vi "Check Linux Partition Size.vi"(8 "Error In":errorcluster, 10 "Warnings":T1[](array[typedef]), 11 "Install LV Data":T2={"SSH Session"=refnum, "Status Log"="", "Detailed Log"="", "Credentials"={"Hostname or IP"="192.168.7.2", "Username"="root", "Password"=""}, "Target Info"={"OS Version"="", "CPU"="", "Systemd Version"="", "Internet Access"=FALSE, "Device Type"="", "LV Installed Ver"="", "LV Available Ver"="", "LV Upgrade Available"=FALSE, "Hostname"="", "NIC Info"=[]}, "Reboot Required?"=FALSE}) -> (0 "Error Out":errorcluster, 2 "Warnings":T1[](array[typedef]), 3 "Install LV Data":T2={"SSH Session"=refnum, "Status Log"="", "Detailed Log"="", "Credentials"={"Hostname or IP"="192.168.7.2", "Username"="root", "Password"=""}, "Target Info"={"OS Version"="", "CPU"="", "Systemd Version"="", "Internet Access"=FALSE, "Device Type"="", "LV Installed Ver"="", "LV Available Ver"="", "LV Upgrade Available"=FALSE, "Hostname"="", "NIC Info"=[]}, "Reboot Required?"=FALSE})   [LabVIEW 2020, in "LMH-LINX.lvlib"]
uses:
  LMH-LINX.lvlib
  Install LV Data.ctl
  Target Info.ctl
  NIC Info.ctl
  NIC Mode.ctl
  Target Compatibility Warnings.ctl
  BBB Expand File System.vi
  <vilib>/regexp/Match Regular Expression.xnode
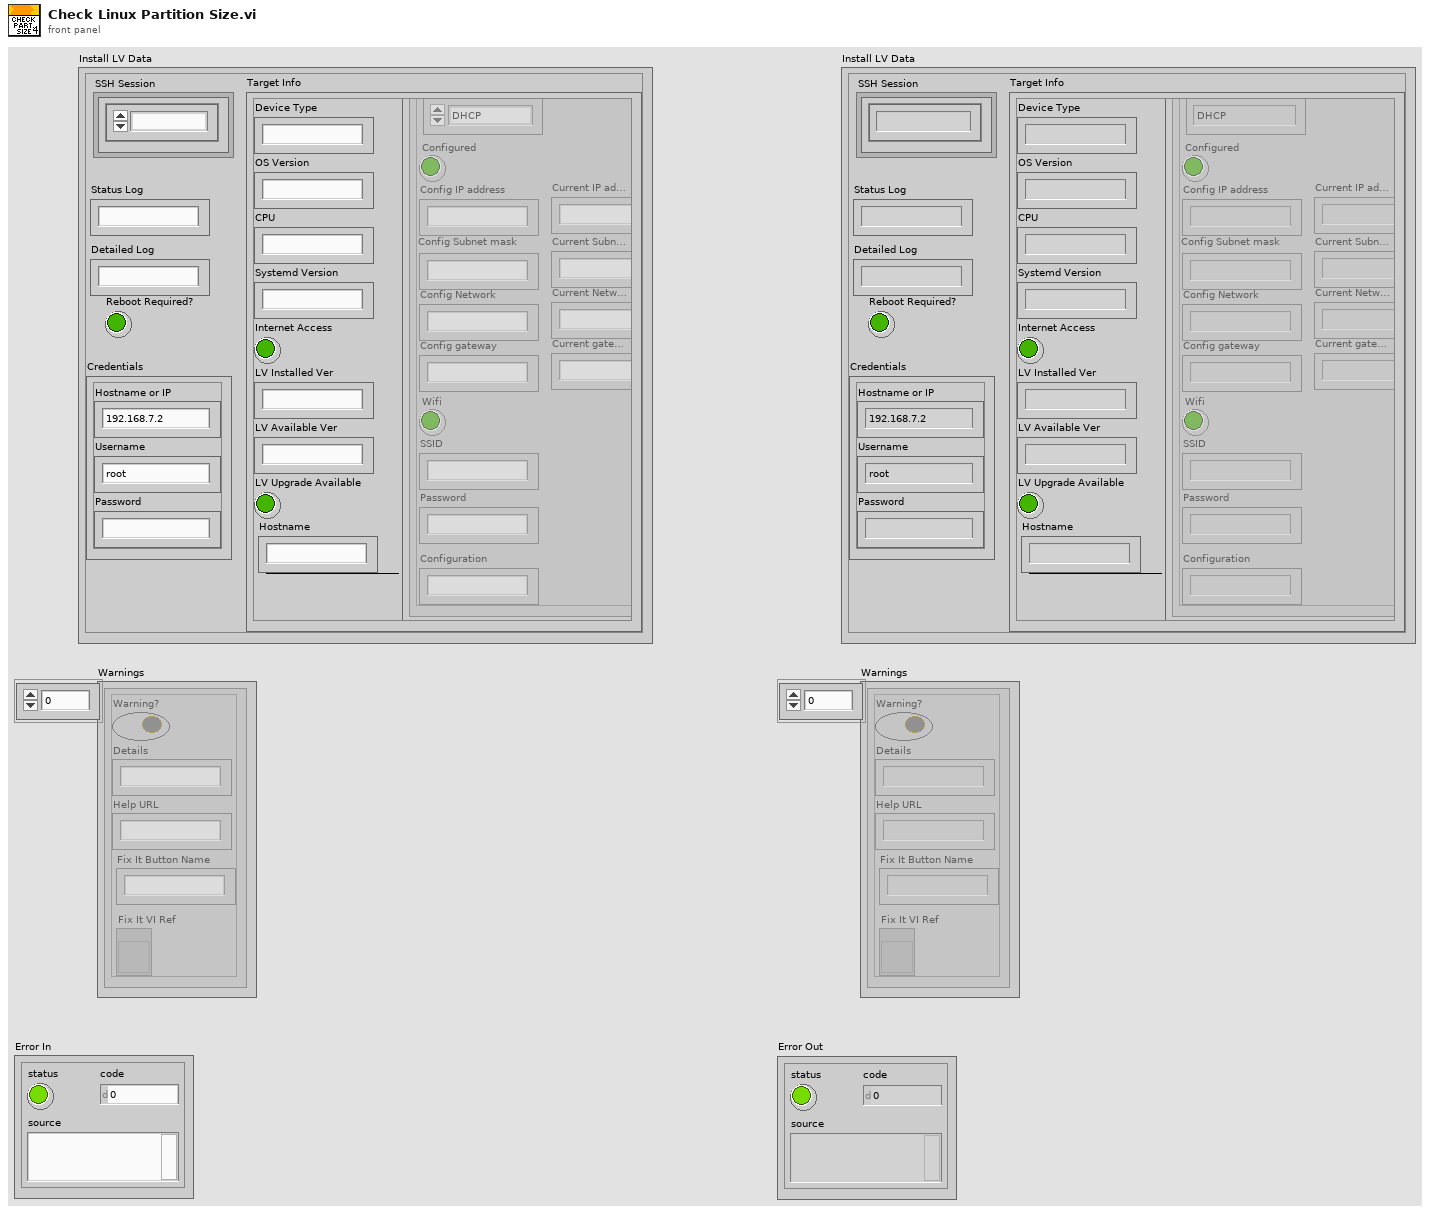
[diagram p1: front panel]
types:
  T1 = typedef "LMH-LINX.lvlib/Target Compatibility Warnings.ctl" = cluster{"Warning?":bool, "Details":string, "Help URL":string, "Fix It Button Name":string, "Fix It VI Ref":refnum<vi>}
  T2 = typedef "LMH-LINX.lvlib/Install LV Data.ctl" = cluster{"SSH Session":refnum<k1>, "Status Log":string, "Detailed Log":string, "Credentials":cluster{"Hostname or IP":string, "Username":string, "Password":string}, "Target Info":T3, "Reboot Required?":bool}
  T3 = typedef "LMH-LINX.lvlib/Target Info.ctl" = cluster{"OS Version":string, "CPU":string, "Systemd Version":string, "Internet Access":bool, "Device Type":string, "LV Installed Ver":string, "LV Available Ver":string, "LV Upgrade Available":bool, "Hostname":string, "NIC Info":T4[]}
  T4 = typedef "LMH-LINX.lvlib/NIC Info.ctl" = cluster{"Name":string, "NIC Mode":T5, "Configured":bool, "Config IP address":string, "Config Subnet mask":string, "Config Network":string, "Config gateway":string, "Wifi":bool, "SSID":string, "Password":string, "Configuration":string, "Current IP address":string, "Current Subnet mask":string, "Current gateway":string, "Current Network":string}
  T5 = typedef "LMH-LINX.lvlib/NIC Mode.ctl" = enum16{"DHCP", "Static", "Loopback"}
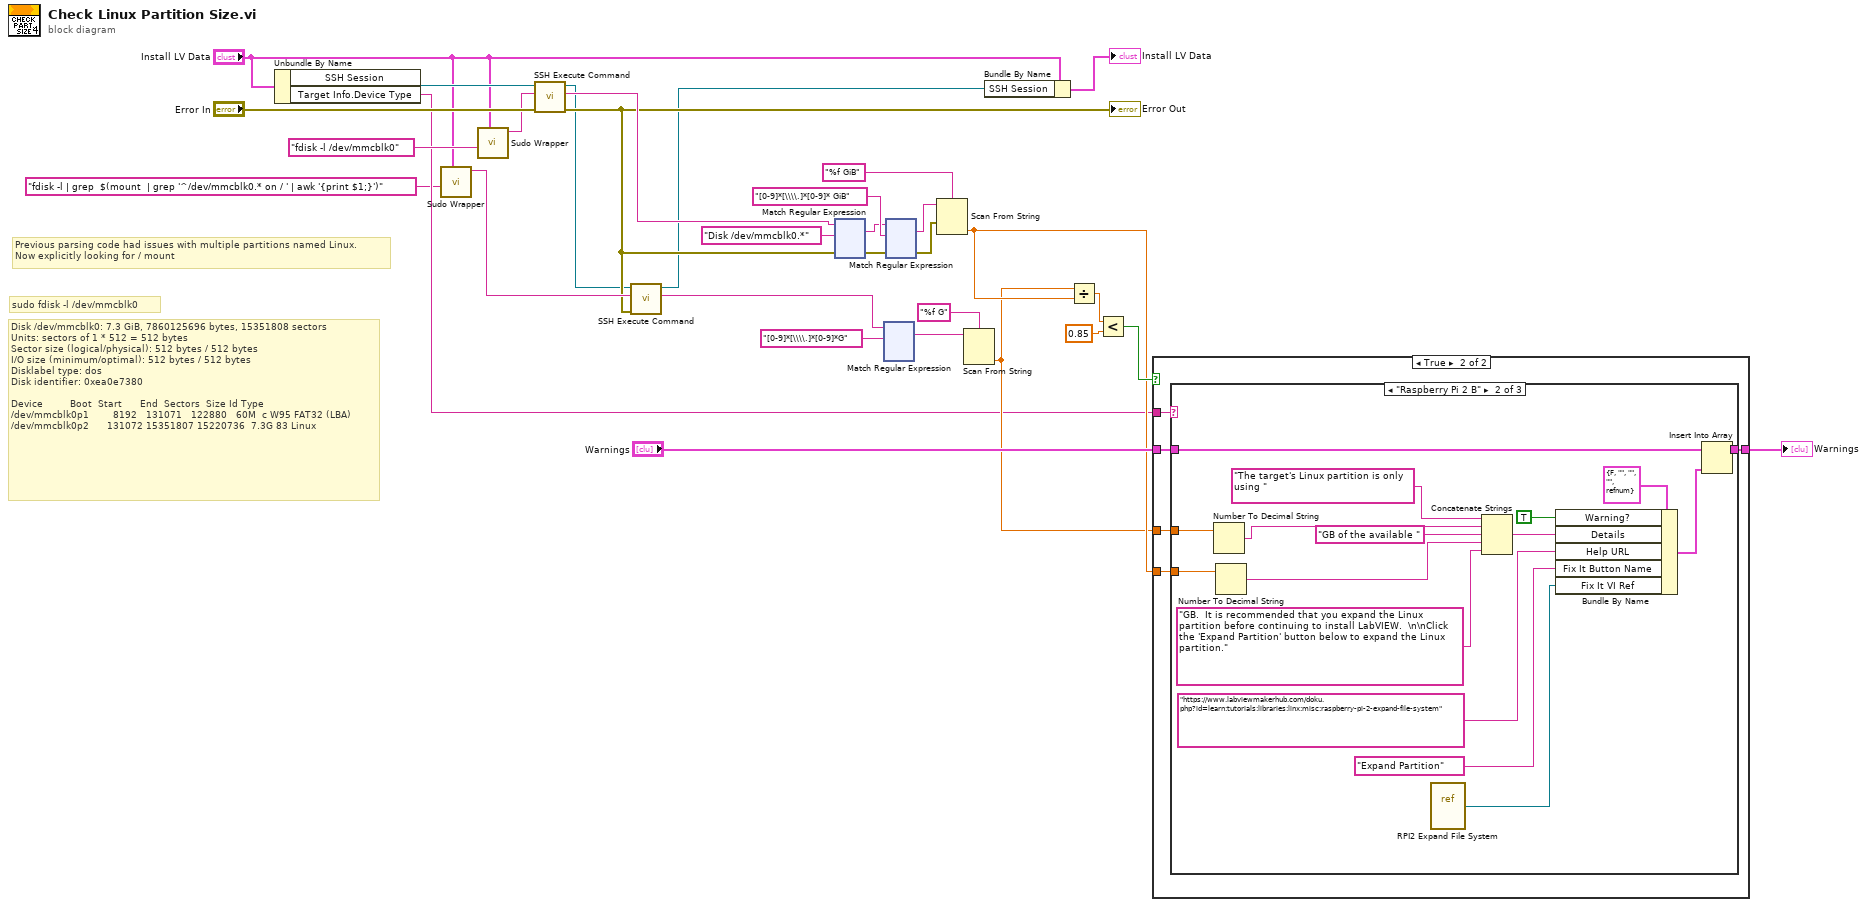
[diagram p0: block diagram]
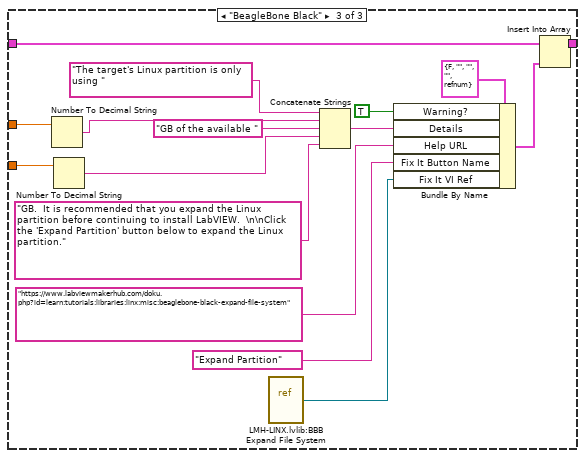
[diagram p4: hidden frame]
diagram:
  # "Previous parsing code had issues with multiple partitions named Linux.\nNow explicitly looking for / mount"
  # "sudo fdisk -l /dev/mmcblk0"
  # "Disk /dev/mmcblk0: 7.3 GiB, 7860125696 bytes, 15351808 sectors\nUnits: sectors of 1 * 512 = 512 bytes\nSector size (logical/physical): 512 bytes / 512 bytes\nI/O size (minimum/optimal): 512 bytes / 512 bytes\nDisklabel type: dos\nDisk identifier: 0xea0e7380\n\nDevice         Boot  Start      End  Sectors  Size Id Type\n/dev/mmcblk0p1        8192   131071   122880   60M  c W95 FAT32 (LBA)\n/dev/mmcblk0p2      131072 15351807 15220736  7.3G 83 Linux"
  n1 = Unbundle By Name("Install LV Data") -> ("SSH Session"=w31:refnum<k1>, "Target Info.Device Type"=w8:string)
  n2 = call "Sudo Wrapper.vi"("Install LV Data"="Install LV Data", "comand string"="fdisk -l | grep  $(mount  | grep '^/dev/mmcblk0.* on / ' | awk '{print $1;}')") -> ("combined command string"=w7:string)  [unwired: 9 in]
  n3 = call "Sudo Wrapper.vi"("Install LV Data"="Install LV Data", "comand string"="fdisk -l /dev/mmcblk0") -> ("combined command string"=w9:string)  [unwired: 9 in]
  n4 = call "SSH Execute Command.vi"("Error In"="Error In", "Command"=w9, "SSH Session"=w31) -> ("Error Out"=w5:errorcluster, "Std Out"=w20:string, "SSH Session"=w3:refnum<k1>)  [unwired: 6 in]
  "Error Out" <- w5
  n5 = call "SSH Execute Command.vi"("Error In"=w5, "Command"=w7, "SSH Session"=w3) -> ("Std Out"=w4:string, "SSH Session"=w2:refnum<k1>)  [unwired: 6 in, 1 out]
  n6 = xnode "Match Regular Expression"("input string"=w20, "regular expression"="Disk /dev/mmcblk0.*" ("String"), "error in"=w5) -> ("whole match"=w25:string, "error out"=w28:errorcluster)  [unwired: 3 in, 3 out]
  n7 = xnode "Match Regular Expression"("input string"=w4, "regular expression"="[0-9]*[\\\\.]*[0-9]*G" ("String")) -> ("whole match"=w22:string)  [unwired: 4 in, 4 out]
  n8 = xnode "Match Regular Expression"("input string"=w25, "regular expression"="[0-9]*[\\\\.]*[0-9]* GiB" ("String"), "error in"=w28) -> ("whole match"=w26:string, "error out"=w17:errorcluster)  [unwired: 3 in, 3 out]
  n9 = Scan From String(format string="%f GiB", input string=w26, error in=w17) -> (output 1=w13:dbl)  [unwired: 2 in, 3 out]
  n10 = Scan From String(format string="%f G", input string=w22) -> (output 1=w12:dbl)  [unwired: 3 in, 3 out]
  n11 = Bundle By Name(cluster="Install LV Data", "SSH Session"=w2) -> (→"Install LV Data":T2)
  n12 = Divide(x=w12, y=w13) -> (x/y=w19:dbl)
  n13 = Less?(x=w19, y=0.85) -> (x < y?=w14:bool)
  n14 = case shown="True" w14 {
    tunnel: "Warnings" -> [w32 w37]
    tunnel: [w32 w36] -> w15
    tunnel: w12 -> [_ w35]
    tunnel: w13 -> [_ w34]
    tunnel: w8 -> [_ w33]
    frame False {
    }
    frame True {
      n15 = case shown="\"Raspberry Pi 2 B\"" w33 {
        tunnel: w37 -> [w38 w49 w65]
        tunnel: [w38 w48 w64] -> w36
        tunnel: w35 -> [_ w47 w63]
        tunnel: w34 -> [_ w41 w57]
        frame "False", Default {
        }
        frame "Raspberry Pi 2 B" {
          n16 = Number To Decimal String(number=w47) -> (decimal integer string=w46:string)  [unwired: 1 in]
          n17 = Number To Decimal String(number=w41) -> (decimal integer string=w44:string)  [unwired: 1 in]
          n18 = vi-ref "RPI2 Expand File System.vi"() -> (w39:refnum<vi>)
          n19 = Concatenate Strings("The target's Linux partition is only using ", w46, "GB of the available " ("string"), w44, "GB.  It is recommended that you expand the Linux partition before continuing to install LabVIEW.  \n\nClick the 'Expand Partition' button below to expand the Linux partition." ("string")) -> (w50:string)
          n20 = Bundle By Name(cluster=T1 {"Warning?"=FALSE, "Details"="", "Help URL"="", "Fix It Button Name"="", "Fix It VI Ref"=refnum} ("Target Compatibility Warnings"), "Warning?"=TRUE ("Can Continue?"), "Details"=w50, "Help URL"="https://www.labviewmakerhub.com/doku.php?id=learn:tutorials:libraries:linx:misc:raspberry-pi-2-expand-file-system" ("string"), "Fix It Button Name"="Expand Partition" ("string"), "Fix It VI Ref"=w39) -> (w51:T1)
          n21 = Insert Into Array(array=w49, new element=w51) -> (w48:T1[])  [unwired: 1 in]
        }
        frame "BeagleBone Black" {
          n22 = Number To Decimal String(number=w63) -> (decimal integer string=w62:string)  [unwired: 1 in]
          n23 = Number To Decimal String(number=w57) -> (decimal integer string=w60:string)  [unwired: 1 in]
          n24 = vi-ref "LMH-LINX.lvlib:BBB Expand File System.vi"() -> (w55:refnum<vi>)
          n25 = Concatenate Strings("The target's Linux partition is only using ", w62, "GB of the available " ("string"), w60, "GB.  It is recommended that you expand the Linux partition before continuing to install LabVIEW.  \n\nClick the 'Expand Partition' button below to expand the Linux partition." ("string")) -> (w66:string)
          n26 = Bundle By Name(cluster=T1 {"Warning?"=FALSE, "Details"="", "Help URL"="", "Fix It Button Name"="", "Fix It VI Ref"=refnum} ("Target Compatibility Warnings"), "Warning?"=TRUE ("Can Continue?"), "Details"=w66, "Help URL"="https://www.labviewmakerhub.com/doku.php?id=learn:tutorials:libraries:linx:misc:beaglebone-black-expand-file-system" ("string"), "Fix It Button Name"="Expand Partition" ("string"), "Fix It VI Ref"=w55) -> (w67:T1)
          n27 = Insert Into Array(array=w65, new element=w67) -> (w64:T1[])  [unwired: 1 in]
        }
      }
    }
  }
  "Warnings" <- w15
